vi "Get Current Sheet.vi"(8 "error in (no error)":errorcluster, 11 "MS-Excel in":refnum<class "MS-Excel.lvclass">) -> (0 "error out":errorcluster, 2 "Sheet Ref":refnum<k24>, 3 "MS-Excel out":refnum<class "MS-Excel.lvclass">)   [LabVIEW 2020, in "LabVIEW NPOI.lvlib" / "MS-Excel.lvclass"]
doc: "Returns a reference, in <b>Sheet Ref</b>, to the active worksheet of the associated workbook to the <b>Document</b>."
uses:
  MS-Excel.lvclass
  D:/Benjamin/Documents/Perso/Code/WC/LabVIEW_NPOI/lib/NPOI 2.1.1/NPOI.dll
  lib/NPOI 2.1.1/NPOI.dll
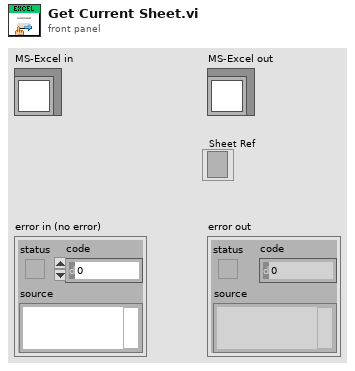
[diagram p1: front panel]
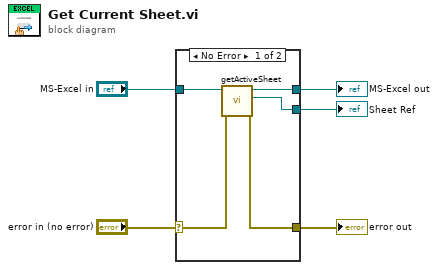
[diagram p0: block diagram]
diagram:
  n1 = case shown="No Error" "error in (no error)" {
    selector: "error in (no error)" -> [w7 w12]
    tunnel: [w6 w12] -> w4
    tunnel: [w9 w11] -> w2
    tunnel: "MS-Excel in" -> [w10 w11]
    tunnel: [w8 _] -> w1
    frame No Error {
      n2 = call-dynamic "getActiveSheet.vi"("error in (no error)"=w7, "MS-Excel in"=w10) -> ("error out"=w6:errorcluster, "Sheet Ref"=w8:refnum<k24>, "MS-Excel out"=w9:refnum<class "MS-Excel.lvclass">)  [unwired: 6 in, 1 out]
    }
    frame Error {
    }
  }
  "error out" <- w4
  "MS-Excel out" <- w2
  "Sheet Ref" <- w1
